vi "OTA Example 1.vi"(8 "Error In":errorcluster) -> (0 "Error Out":errorcluster)   [LabVIEW 2014]
uses:
  ESP8266-Wifi-Wrapper/ESP8266 WiFi Wrapper.lvlib
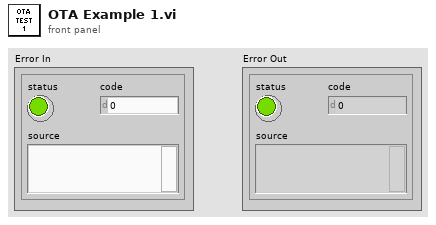
[diagram p1: front panel]
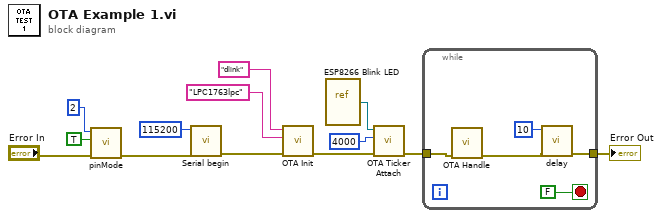
[diagram p0: block diagram]
diagram:
  n1 = call <vilib>:"pinMode.vi"("Error In"="Error In", "output?"=TRUE, "pin number"=2) -> ("Error Out"=w4:errorcluster)  [unwired: 8 in]
  n2 = call <vilib>:"Serial begin.vi"("Error In"=w4, "speed (Bd)"=115200) -> ("Error Out"=w12:errorcluster)  [unwired: 9 in]
  n3 = call <vilib>:"OTA Init.vi"("Error In"=w12, "password"="LPC1763lpc" ("ssid"), "ssid"="dlink") -> ("Error Out"=w9:errorcluster)  [unwired: 8 in]
  n4 = vi-ref "ESP8266 Blink LED.vi"() -> (w8:refnum<vi>)
  n5 = call <vilib>:"OTA Ticker Attach.vi"("Error In"=w9, "interval (sec.)"=u32 4000, "VI Refnum"=w8) -> ("Error Out"=w6:errorcluster)  [unwired: 8 in]
  n6 = while {
    tunnel: w6 -> [w18]
    tunnel: [w15] -> w7
    stop <- FALSE stop-if-true
    n7 = call "OTA Handle.vi"("Error In"=w18) -> ("Error Out"=w16:errorcluster)  [unwired: 10 in]
    n8 = call <vilib>:"delay.vi"("Error In"=w16, "time (ms)"=10) -> ("Error Out"=w15:errorcluster)  [unwired: 9 in]
  }
  "Error Out" <- w7
